vi "Change Copy LLB to NI VeriStand.vi"(8 "error in (no error)":errorcluster, 10 "Copy .LLB to ... path":path, 11 "CD Wizard - Internal Data":T1) -> (0 "error out":errorcluster)   [LabVIEW 2015]
doc: "Change the block diagram of \"Copy .LLB to NI VeriStand dir\" accoding to the custom device name and the execution mode."
uses:
  TypDef/CD Wizard - Internal data.ctl
  TypDef/CD Wizard - Execution Mode.ctl
  TypDef/CD Wizard - Extra Page Name and GUID.ctl
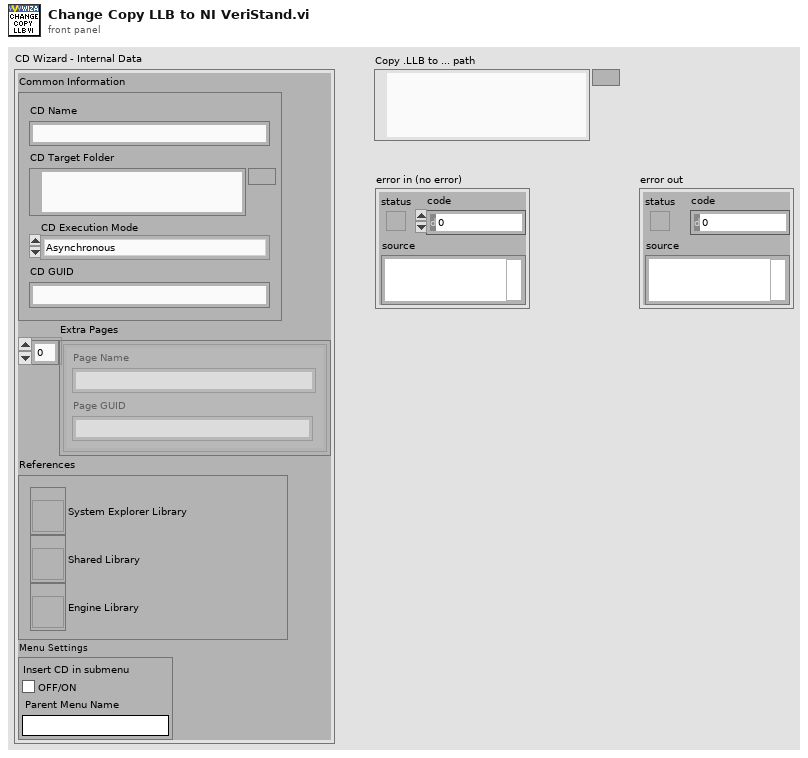
[diagram p1: front panel]
types:
  T1 = typedef "CD Wizard - Internal data.ctl" = cluster{"Common Information":cluster{"CD Name":string, "CD Target Folder":path, "CD Execution Mode":T2, "CD GUID":string}, "Extra Pages":T3[], "References":cluster{"System Explorer Library":refnum<vi>, "Shared Library":refnum<vi>, "Engine Library":refnum<vi>}, "Menu Settings":cluster{"Insert CD in submenu":bool, "Parent Menu Name":string}}
  T2 = typedef "CD Wizard - Execution Mode.ctl" = enum16{"Asynchronous", "Inline HW Interface", "Inline Model Interface", "Inline Timing and Sync", "Asynchronous Timing and Sync"}
  T3 = typedef "CD Wizard - Extra Page Name and GUID.ctl" = cluster{"Page Name":string, "Page GUID":string}
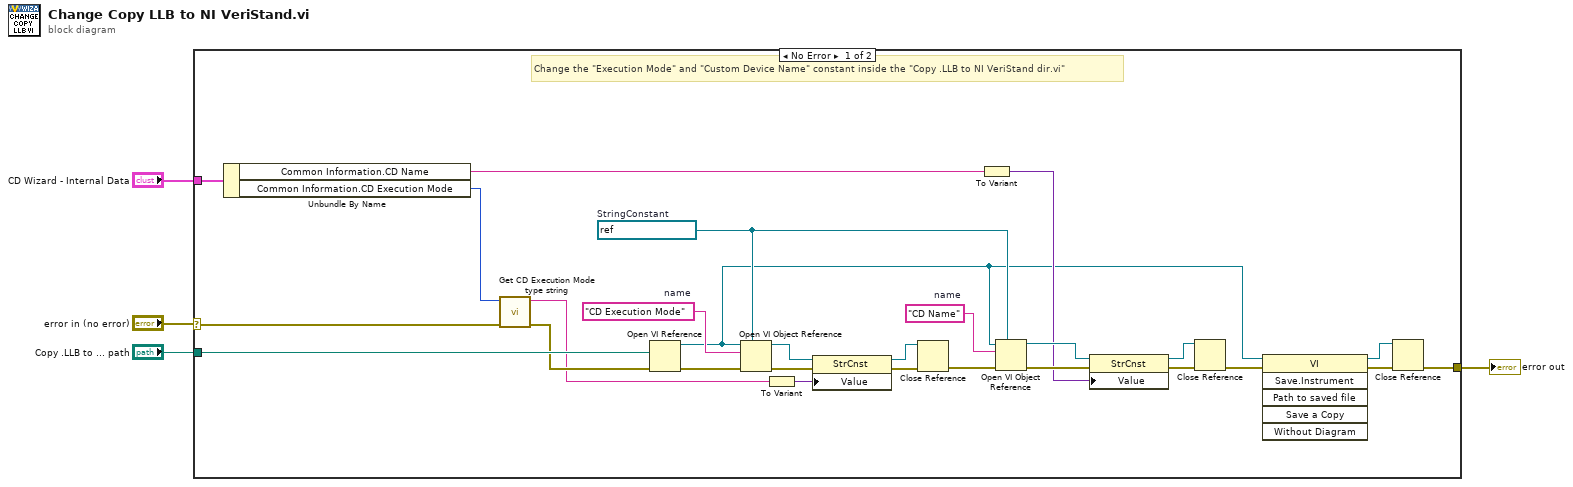
[diagram p0: block diagram]
diagram:
  n1 = case shown="No Error" "error in (no error)" {
    selector: "error in (no error)" -> [w8 w32]
    tunnel: [w13 w32] -> w3
    tunnel: "CD Wizard - Internal Data" -> [w12 _]
    tunnel: "Copy .LLB to ... path" -> [w10 _]
    frame No Error {
      w23 = "CD Name"  # name
      w31 = "CD Execution Mode"  # name
      w24 = refnum<vi> refnum  # StringConstant
      # "Change the \"Execution Mode\" and \"Custom Device Name\" constant inside the \"Copy .LLB to NI VeriStand dir.vi\""
      n2 = Unbundle By Name(w12) -> ("Common Information.CD Name"=w9:string, "Common Information.CD Execution Mode"=w6:T2)
      n3 = call "Get CD Execution Mode type string.vi"("error in (no error)"=w8, "CD Execution Mode"=w6) -> ("error out"=w7:errorcluster, "Execution Mode type"=w5:string)  [unwired: 8 in]
      n4 = Open VI Reference(vi path=w10, error in (no error)=w7) -> (vi reference=w15:refnum<vi>, error out=w11:errorcluster)  [unwired: 4 in]
      n5 = Open VI Object Reference(7:w24, 8:w11, 10:w31, 11:w15) -> (0:w30:errorcluster, 3:w27:refnum<vi>)
      n6 = To Variant(anything=w5) -> (Variant=w26:variant)
      n7 = property class="StrCnst"(reference=w27, error in=w30, "Value"=w26) -> (reference out=w29:refnum<vi>, error out=w28:errorcluster)
      n8 = Close Reference(reference=w29, error in (no error)=w28) -> (error out=w25:errorcluster)
      n9 = To Variant(anything=w9) -> (Variant=w18:variant)
      n10 = Open VI Object Reference(7:w24, 8:w25, 10:w23, 11:w15) -> (0:w22:errorcluster, 3:w21:refnum<vi>)
      n11 = property class="StrCnst"(reference=w21, error in=w22, "Value"=w18) -> (reference out=w16:refnum<vi>, error out=w17:errorcluster)
      n12 = Close Reference(reference=w16, error in (no error)=w17) -> (error out=w14:errorcluster)
      n13 = invoke class="VI" method="Save.Instrument"(reference=w15, error in=w14) -> (reference out=w20:refnum<vi>, error out=w19:errorcluster)  [unwired: 4 in, 4 out]
      n14 = Close Reference(reference=w20, error in (no error)=w19) -> (error out=w13:errorcluster)
    }
    frame Error {
      # "Output default values."
    }
  }
  "error out" <- w3
